vi "Handle Last Ack Core.vi"(4 "error in (no error)":errorcluster, 6 "Last Ack":refnum<class "Last Ack.lvclass">, 7 "Process Model in":refnum<class "Process Model.lvclass">) -> (0 "error out":errorcluster, 3 "Process Model out":refnum<class "Process Model.lvclass">)   [LabVIEW 2017, in "Process Model.lvlib" / "Process Model.lvclass"]
doc: "(<B>Filename</B>: Actor Framework.lvlib:Actor.lvclass:Handle Last Ack Core.vi)\n\nDefines how the caller actor responds to the Last Ack message from a nested actor. The Last Ack message is the final message a nested actor sends to its caller before it shuts down. The message contains information about the final state of the nested actor.\n\nBy default, this method does nothing except return any error the nested actor sent. A descendant class may override this method to define behavior."
uses:
  <vilib>/gpm_packages/@cs/Car wash/Process Model/Process Model/Process Model.lvclass
  <vilib>/ActorFramework/LastAck/Last Ack.lvclass
  <vilib>/gpm_packages/@cs/Carwash/Source/iProcess Step Model/iProcess Step Model/iProcess Step Model.lvclass
  <vilib>/ActorFramework/Actor/Actor.lvclass
  <vilib>/ActorFramework/Message Enqueuer/Message Enqueuer.lvclass
  <vilib>/gpm_packages/@cs/Car wash/iProcess Model/iProcess Model/iProcess Model.lvclass
  C:/Program Files/National Instruments/LabVIEW 2017/vi.lib/gpm_packages/@cs/Car wash/iProcess Model/iProcess Model/iProcess Model.lvclass
  C:/Program Files/National Instruments/LabVIEW 2017/vi.lib/gpm_packages/@cs/mva-core/Source/IModel/IModel/IModel.lvclass
  C:/Program Files/National Instruments/LabVIEW 2017/vi.lib/gpm_packages/@cs/mva-core/Source/IObserver/IObserver/IObserver.lvclass
  C:/Program Files/National Instruments/LabVIEW 2017/vi.lib/ActorFramework/Actor/Actor.lvclass
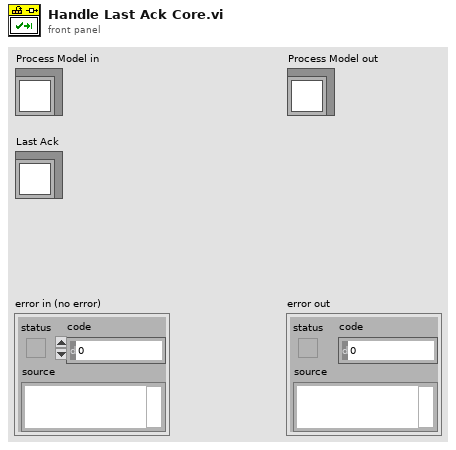
[diagram p1: front panel]
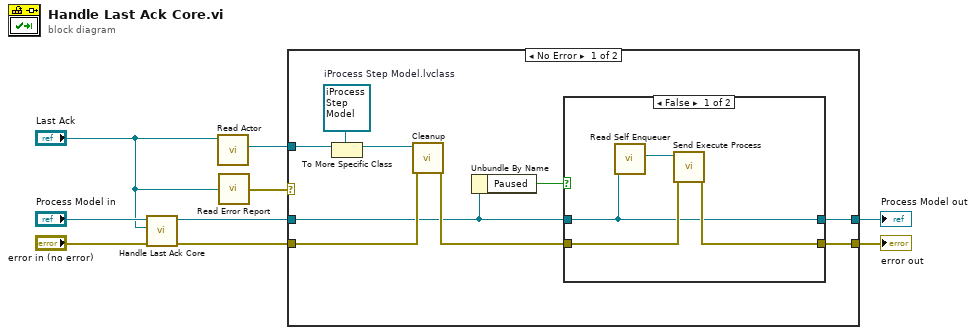
[diagram p0: block diagram]
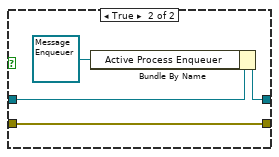
[diagram p2: hidden frame]
diagram:
  n1 = call-parent "Handle Last Ack Core.vi"("error in (no error)"="error in (no error)", "Last Ack"="Last Ack", "IModel in"="Process Model in") -> ("error out"=w5:errorcluster, "IModel out"=w3:refnum<class "Process Model.lvclass">)  [unwired: 3 in]
  n2 = call <vilib>:"Read Actor.vi"("Last Ack"="Last Ack") -> ("Actor"=w6:refnum<class "Actor.lvclass">)  [unwired: 10 in]
  n3 = call <vilib>:"Read Error Report.vi"("Last Ack"="Last Ack") -> ("error report"=w1:errorcluster)
  n4 = case shown="No Error" w1 {
    selector: w1 -> [_ w27]
    tunnel: w6 -> [w18 _]
    tunnel: w5 -> [w16 _]
    tunnel: [w14 w27] -> w4
    tunnel: w3 -> [w13 w28]
    tunnel: [w12 w28] -> w2
    frame No Error {
      w10 = refnum<class "iProcess Step Model.lvclass"> refnum  # iProcess Step Model.lvclass
      n5 = To More Specific Class(target class=w10, reference=w18) -> (specific class reference=w17:refnum<class "iProcess Step Model.lvclass">)  [unwired: 1 in, 1 out]
      n6 = call-dynamic "Cleanup.vi"("error in (no error)"=w16, "iProcess Step Model in"=w17) -> ("error out"=w15:errorcluster)  [unwired: 8 in, 1 out]
      n7 = Unbundle By Name(w13) -> ("Paused"=w11:bool)
      n8 = case shown="False" w11 {
        tunnel: w15 -> [w21 w26]
        tunnel: [w20 w26] -> w14
        tunnel: w13 -> [w19 w25]
        tunnel: [w19 w24] -> w12
        frame False {
          n9 = call <vilib>:"Read Self Enqueuer.vi"("Actor"=w19) -> ("Self Enqueuer"=w22:refnum<class "Message Enqueuer.lvclass">)  [unwired: 10 in]
          n10 = call <vilib>:"Send Execute Process.vi"("error in (no error)"=w21, "Message Enqueuer"=w22) -> ("error out"=w20:errorcluster)  [unwired: 8 in, 1 out]
        }
        frame True {
          n11 = Bundle By Name(cluster=w25, "Active Process Enqueuer"=refnum<class "Message Enqueuer.lvclass"> refnum) -> (w24:refnum<class "Process Model.lvclass">)
        }
      }
    }
    frame Error {
    }
  }
  "Process Model out" <- w2
  "error out" <- w4
